vi "Memory Management.Handle Return.vi"(8 "error in (no error)":errorcluster, 11 "return":i32) -> (0 "error out":errorcluster)   [LabVIEW 2016, in "VeriStand Data.lvlib"]
uses:
  VeriStand Data.lvlib
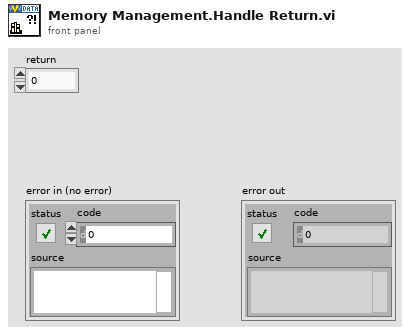
[diagram p1: front panel]
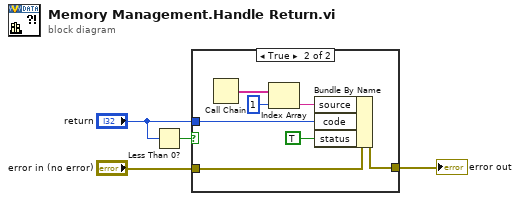
[diagram p0: block diagram]
diagram:
  n1 = Less Than 0?(x="return") -> (x < 0?=w4:bool)
  n2 = case shown="True" w4 {
    tunnel: "return" -> [_ w8]
    tunnel: [w5 w10] -> w2
    tunnel: "error in (no error)" -> [w5 w6]
    frame False {
    }
    frame True {
      n3 = Call Chain() -> (call chain=w11:string[])
      n4 = Index Array(array=w11, index=1) -> (element=w7:string)
      n5 = Bundle By Name(cluster=w6, "source"=w7, "code"=w8, "status"=TRUE) -> (w10:errorcluster)
    }
  }
  "error out" <- w2
